vi "PH_Sound.Soundtest.vi"(5 "error in":errorcluster) -> (19 "Device error":errorcluster)   [LabVIEW 2014, in "PH_Sound.lvlib"]
doc: "By this VI a ross relais can be monitored and switched. \n\nThe indicators \"CLOSED\", \"OPEN\" and \"SWITCH STATE\" show the value of the Beckhoff-Tag: blue indicates bad tag status reference problems, darkgreen false and lightgreen on. If everything is working fine, \"CLOSED\" and \"SWITCH STATE\" should show the same value, while \"OPEN\" has the opposite value. \n\nThe oval button switches the ross relais. It should be in the same state as the \"SWITCH STATE\" indicator. \n\n\"EXIT\" closes the front panel (GUI), while \"Delete Instance\" disconnects and removes the instance from the PCS.\n\nThis VI has no machine safety relevant logig: there is neither a check of internal conclict nor with other objects, for example conflict with other ross relais. Therefore it must be handled with care and should be operated by well educated operators only. It is forseen exclusively for direct operating and testing of the system. \n\nLicense Agreement for this software:\n\nCopyright (C)\nGesellschaft für Schwerionenforschung, GSI\nPlanckstr. 1\n64291 Darmstadt\nGermany\n\nContact: D.Beck@gsi.de \n\nThis program is free software; you can redistribute it and/or modify it under the terms of the GNU General Public License as published by the Free Software Foundation; either version 2 of the license, or (at your option) any later version.\n\nThis program is distributed in the hope that it will be useful, but WITHOUT ANYW ARRANTY; without even the implied warranty of MERCHANTABILITY or FITNESS FOR A PARTICULAR PURPOSE. See the GNU General License for more details (http://www.gnu.org).\n\nGesellschaft für Schwerionenforschung, GSI\nPlanckstr. 1, 64291 Darmstadt, Germany\nFor all questions and ideas contact: M.Richter@gsi.de, H.Brand@gsi.de or D.Beck@gsi.de.\nLast update: 18-DEC-2002"
uses:
  PH_Sound.lvlib
  PH_Sound.3Oktaves.ctl
panel:
  in  "Play Song":bool
  in  "path":path=path "D:/PCS/Sound/Beeth9th.wav"
  in  "Play Wave":bool
  in  "3 Octaves":T1=130.8 items=["c"=130.8, "cis"=138.6, "d"=146.8, "es"=155.6, "e"=164.8, "f"=174.6, "fis"=185.0, "g"=196.0, "as"=207.6, "a"=220.0, "b"=233.1, "h"=246.9, "c'"=261.6, "cis'"=277.2, "d'"=293.7, "es'"=311.1, "e'"=329.6, "f'"=349.2, "fis'"=370.0, "g'"=392.0, "as'"=415.3, "a'"=440.0, "b'"=466.2, "h'"=493.9, "c''"=523.3, "cis''"=554.4, "d''"=587.3, "es''"=622.3, "e''"=659.3, "f''"=689.5, "fis''"=740.0, "g''"=784.0, "as''"=830.6, "a''"=880.0, "b''"=932.3, "h''"=987.8, "c'''"=1047.0]
  in  "b":bool
  in  "as":bool
  in  "fis":bool
  in  "es":bool
  in  "cis":bool
  in  "h":bool
  in  "a":bool
  in  "g":bool
  in  "f":bool
  in  "e":bool
  in  "d":bool
  in  "c":bool
  in  "b''":bool
  in  "as''":bool
  in  "fis''":bool
  in  "es''":bool
  in  "cis''":bool
  in  "h''":bool
  in  "a''":bool
  in  "g''":bool
  in  "f''":bool
  in  "e''":bool
  in  "d''":bool
  in  "c''":bool
  in  "c'''":bool
  in  "b'":bool
  in  "as'":bool
  in  "fis'":bool
  in  "es'":bool
  in  "cis'":bool
  in  "h'":bool
  in  "a'":bool
  in  "g'":bool
  in  "f'":bool
  in  "e'":bool
  in  "d'":bool
  in  "c'":bool
  in  "Delete":bool
  # "PCS"
  # "3.40"
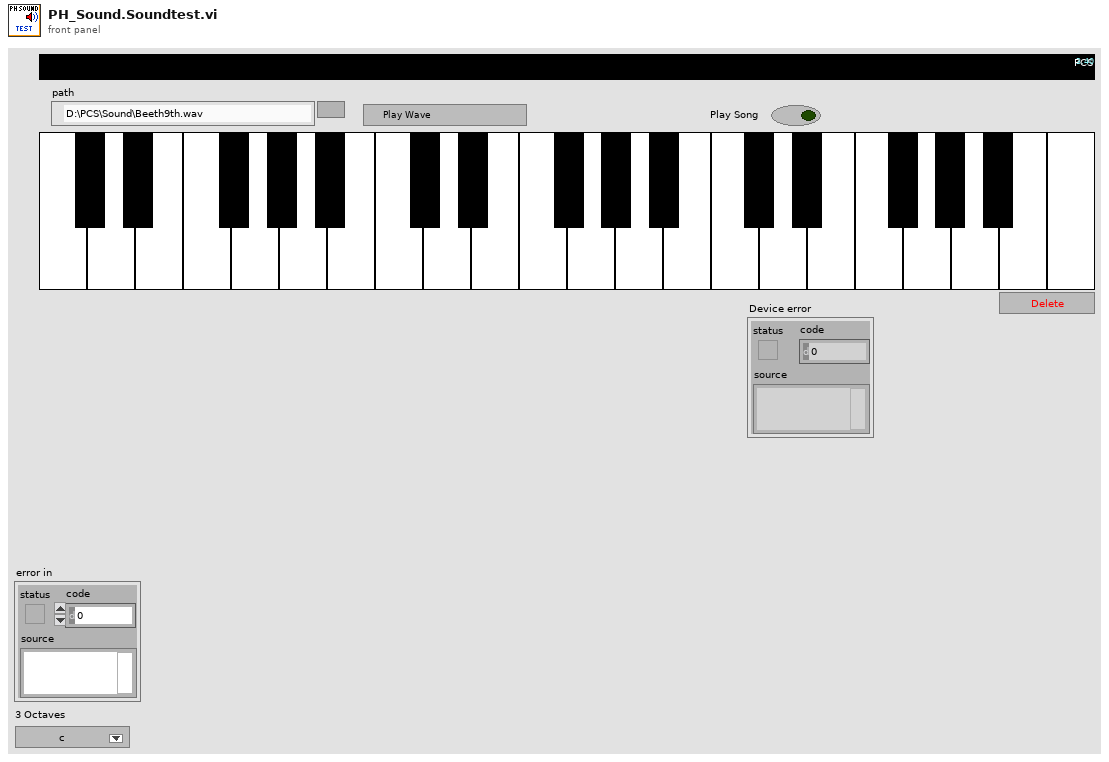
[diagram p1: front panel]
types:
  T1 = typedef "PH_Sound.lvlib/PH_Sound.3Oktaves.ctl" = dbl
  T2 = typedef "LVStringsAndValuesArrayTypeDef_DBL.ctl" = cluster{"String":string, "Value":dbl}[]
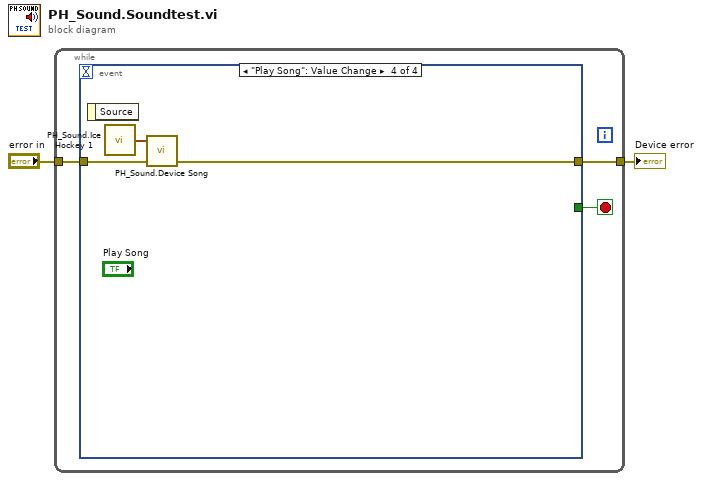
[diagram p0: block diagram]
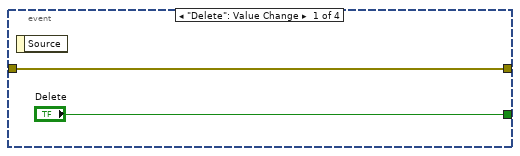
[diagram p2: hidden frame]
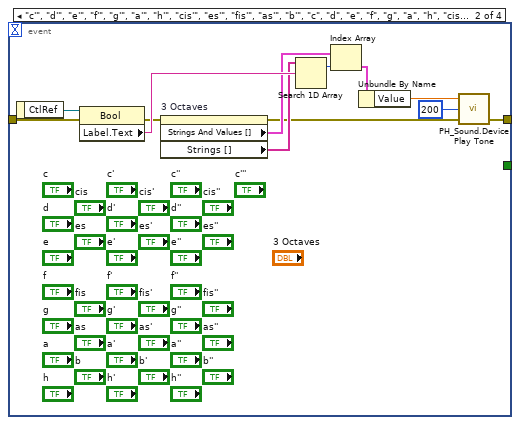
[diagram p3: hidden frame]
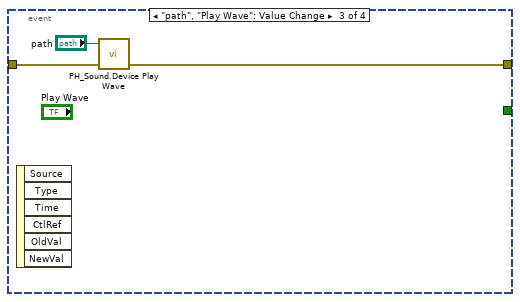
[diagram p4: hidden frame]
diagram:
  n1 = while {
    tunnel: "error in" -> [w4]
    tunnel: [w3] -> w2
    stop <- w5 stop-if-true
    n2 = event shown="[3] \"Play Song\": Value Change" {
      selector: _ -> [_ _ _ _]
      dyn-events: _ -> [_ _ _ _]
      timeout: _ -> [_ _ _ _]
      tunnel: ["Delete" _ _ _] -> w5
      tunnel: w4 -> [w6 w18 w22 w25]
      tunnel: [w6 w11 w21 w24] -> w3
      event "Delete": Value Change {
        n3 = event-data() -> ()  [unwired: 1 in, 1 out]
      }
      event "c'", "d'", "e'", "f'", "g'", "a'", "h'", "cis'", "es'", "fis'", "as'", "b'", "c", "d", "e", "f", "g", "a", "h", "cis", "es", "fis", "as", "b", "c''", "d''", "e''", "f''", "g''", "a''", "h''", "c'''", "cis''", "es''", "fis''", "as''", "b''": Value Change {
        n4 = event-data() -> ("CtlRef"=w19:refnum<vi>)  [unwired: 1 in]
        n5 = property class="Bool"(reference=w19, error in=w18) -> (error out=w12:errorcluster, "Label.Text"=w17:string)  [unwired: 1 out]
        n6 = property on="3 Octaves" class="Ring (strict)"(error in=w12) -> (error out=w8:errorcluster, "Strings And Values []"=w15:T2, "Strings []"=w16:string[])  [unwired: 1 in, 1 out]
        n7 = Search 1D Array(1D array=w16, element=w17) -> (index of element=w14:i32)  [unwired: 1 in]
        n8 = Index Array(array=w15, index=w14) -> (element=w13:cluster{"String":string, "Value":dbl})
        n9 = Unbundle By Name(w13) -> ("Value"=w9:dbl)
        n10 = call "PH_Sound.Device Play Tone.vi"("error in"=w8, "Length [ms]"=200 ("Legth [ms]"), "tone"=w9) -> ("Device error out"=w11:errorcluster)  [unwired: 2 in]
      }
      event "path", "Play Wave": Value Change {
        n11 = event-data() -> ()  [unwired: 1 in, 6 out]
        n12 = call "PH_Sound.Device Play Wave.vi"("error in (no error)"=w22, "path"="path") -> ("Device error out"=w21:errorcluster)  [unwired: 3 in]
      }
      event "Play Song": Value Change {
        n13 = event-data() -> ()  [unwired: 1 in, 1 out]
        n14 = call "PH_Sound.Ice Hockey 1.vi"() -> ("Ice Hockey 1"=w23:cluster{"Tone":dbl, "Beats":i32}[])  [unwired: 1 in]
        n15 = call "PH_Sound.Device Song.vi"("error in (no error)"=w25, "Song"=w23) -> ("error out"=w24:errorcluster)  [unwired: 3 in]
      }
    }
  }
  "Device error" <- w2
